vi "Release Queue.vi"(8 "Error In":errorcluster, 11 "Queue Ref In":refnum<queue>) -> (0 "Error Out":errorcluster)   [LabVIEW 2016, in "SLL QSM.lvlib"]
doc: "Release the Queue Reference"
uses:
  SLL QSM.lvlib
  Typedefs/Queue Type.ctl
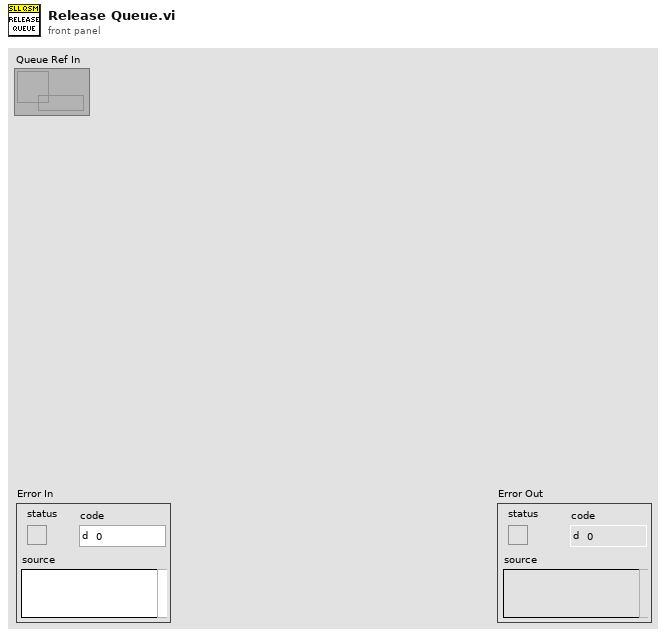
[diagram p1: front panel]
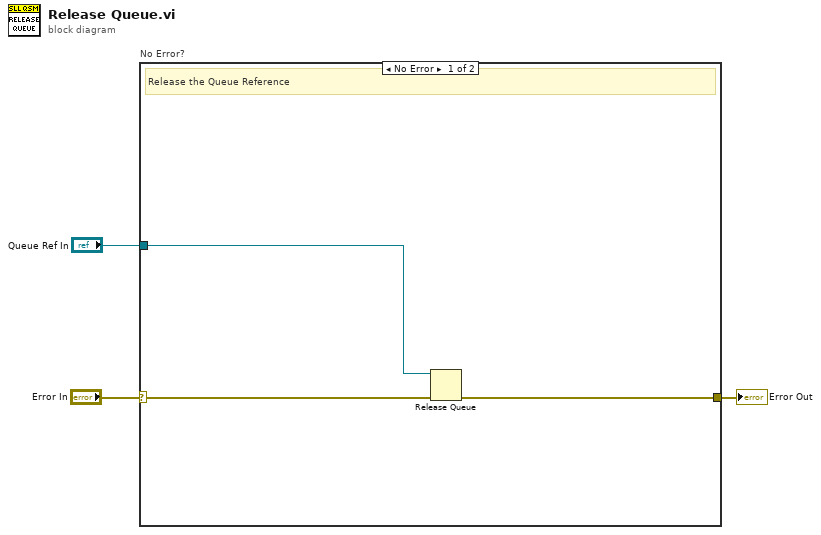
[diagram p0: block diagram]
diagram:
  n1 = case "No Error?" shown="No Error" "Error In" {
    selector: "Error In" -> [w4 w7]
    tunnel: [w6 w7] -> w3
    tunnel: "Queue Ref In" -> [w5 _]
    frame No Error {
      # "Release the Queue Reference"
      n2 = Release Queue(queue=w5, error in (no error)=w4) -> (error out=w6:errorcluster)  [unwired: 1 in, 2 out]
    }
    frame Error {
    }
  }
  "Error Out" <- w3
